vi "mWmotor_STOP.vi"(8 "error in (no error)":errorcluster, 10 "milliseconds to wait":u32=100, 11 "VISA resource name":refnum<visa-resource-name>) -> (0 "error out":errorcluster, 2 "MI buffer":string, 3 "VISA resource name out":refnum<visa-resource-name>)   [LabVIEW 2019]
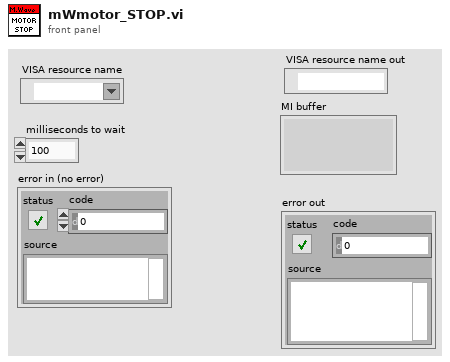
[diagram p1: front panel]
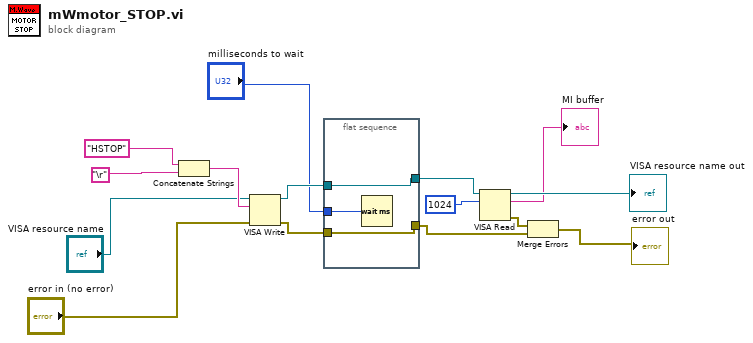
[diagram p0: block diagram]
diagram:
  n1 = Concatenate Strings("HSTOP" ("string"), "\r") -> (w15:string)
  n2 = VISA Write(VISA resource name="VISA resource name", write buffer=w15, error in (no error)="error in (no error)") -> (VISA resource name out=w10:refnum<visa-resource-name>, error out=w11:errorcluster)  [unwired: 1 out]
  n3 = flat-sequence {
    tunnel: [w18] -> w3
    tunnel: w11 -> [w18]
    tunnel: [w17] -> w9
    tunnel: w10 -> [w17]
    tunnel: "milliseconds to wait" -> [w16]
    frame #0 {
      n4 = Wait (ms)(milliseconds to wait=w16) -> ()  [unwired: 1 out]
    }
  }
  n5 = VISA Read(VISA resource name=w9, byte count=u32 1024) -> (VISA resource name out=→"VISA resource name out":refnum<visa-resource-name>, read buffer=→"MI buffer":string, error out=w1:errorcluster)  [unwired: 1 in, 1 out]
  n6 = Merge Errors(w1, w3) -> (→"error out":errorcluster)
